vi "I2C Settings from ini.vi"(7 "Section":string, 8 "error in (no error)":errorcluster, 11 "Protocol_Timing In":T1={"SCL Period (Ticks)"=400, "StartDelay(Ticks)"=1200, "StopDelay(Ticks)"=1200, "PostAddressDelay(Ticks)"=1200, "TransmitDelay(Ticks)"=1000}) -> (0 "error out":errorcluster, 3 "Protocol_Timing Out":T1={"SCL Period (Ticks)"=400, "StartDelay(Ticks)"=1200, "StopDelay(Ticks)"=1200, "PostAddressDelay(Ticks)"=1200, "TransmitDelay(Ticks)"=1000}, 5 "All Tags Exists?":bool)   [LabVIEW 2013]
doc: "Loads the I2C Timing protocol parameters from the ini file."
uses:
  Common/File IO/INI/Read write mode.ctl
  I2C Settings Enum Keys.ctl
  I2C/i2c_Protocol_Timing.ctl
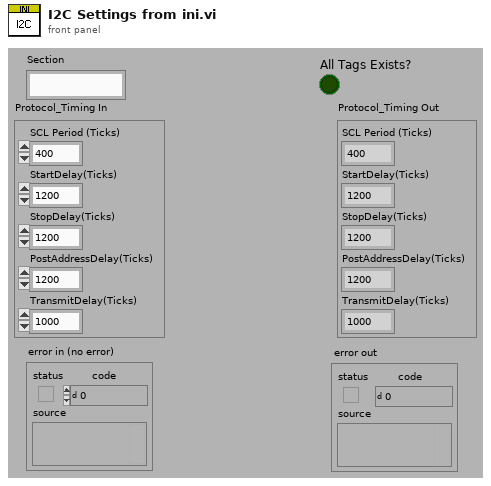
[diagram p1: front panel]
types:
  T1 = typedef "i2c_Protocol_Timing.ctl" = cluster{"SCL Period (Ticks)":u32, "StartDelay(Ticks)":u32, "StopDelay(Ticks)":u32, "PostAddressDelay(Ticks)":u32, "TransmitDelay(Ticks)":u32}
  T2 = typedef "I2C Settings Enum Keys.ctl" = enum16{"SCL Period (Ticks)", "Start Delay (Ticks)", "Stop Delay (Ticks)", "Post Address Delay (Ticks)", "Transmit Delay (Ticks)"}
  T3 = typedef "Read write mode.ctl" = enum16{"Read", "Write"}
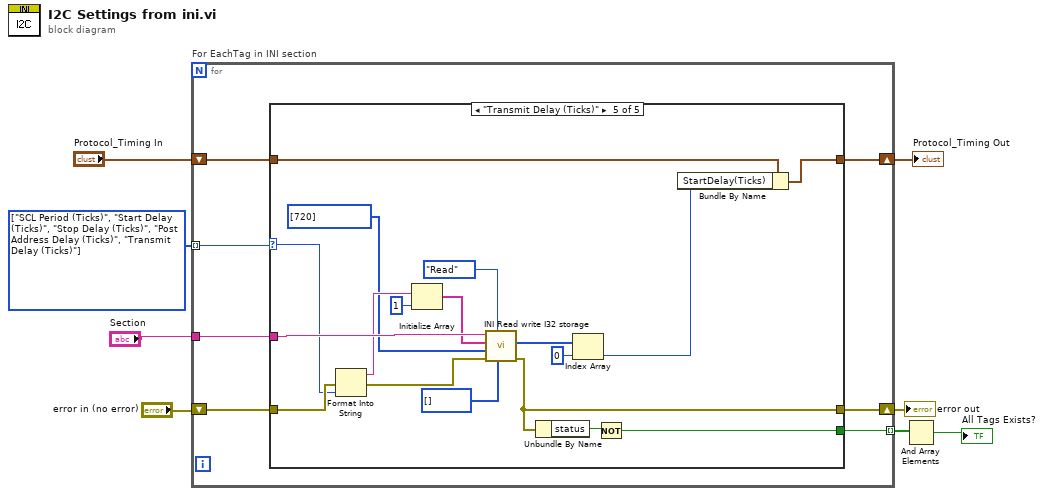
[diagram p0: block diagram]
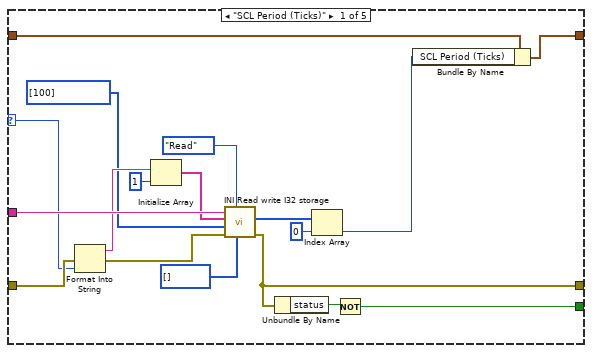
[diagram p2: hidden frame]
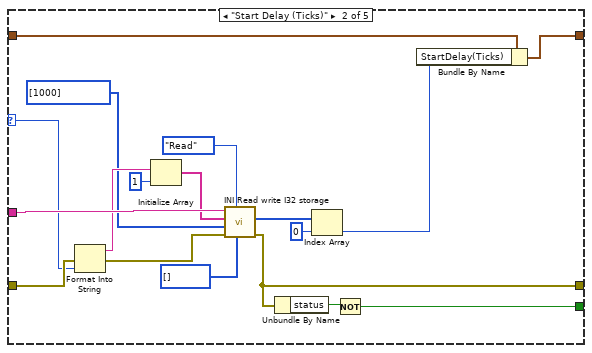
[diagram p3: hidden frame]
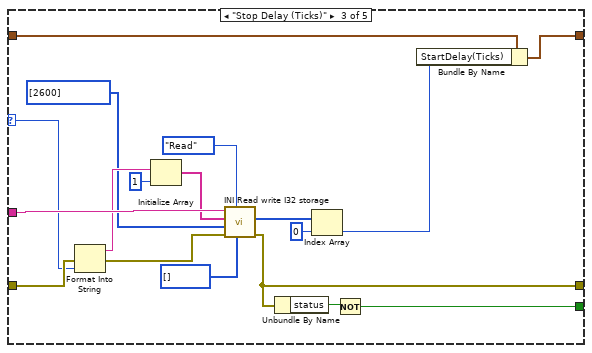
[diagram p4: hidden frame]
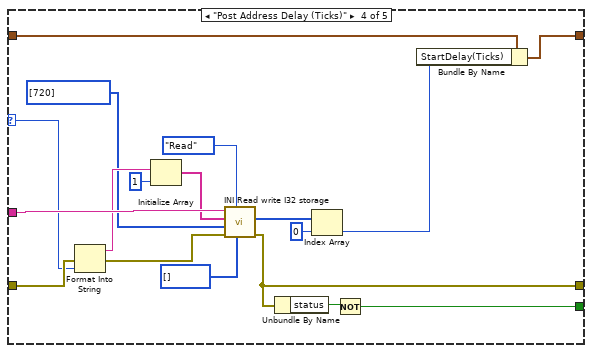
[diagram p5: hidden frame]
diagram:
  w8 = T2[] [enum."SCL Period (Ticks)", enum."Start Delay (Ticks)", enum."Stop Delay (Ticks)", enum."Post Address Delay (Ticks)", enum."Transmit Delay (Ticks)"] items=["SCL Period (Ticks)", "Start Delay (Ticks)", "Stop Delay (Ticks)", "Post Address Delay (Ticks)", "Transmit Delay (Ticks)"]
  n1 = for "For EachTag in INI section" {
    tunnel: "Section" -> [w15]
    tunnel: w8 -> [w14] mode=indexing
    shift-right: [w10] -> w6
    shift-left: "error in (no error)" -> [w12]
    shift-right: [w9] -> w1
    shift-left: "Protocol_Timing In" -> [w13]
    tunnel: [w11] -> w4 mode=indexing
    n2 = case shown="\"Transmit Delay (Ticks)\"" w14 {
      selector: w14 -> [w28 w46 w64 w82 w100]
      tunnel: w15 -> [w32 w50 w68 w86 w104]
      tunnel: w13 -> [w30 w48 w66 w84 w102]
      tunnel: w12 -> [w29 w47 w65 w83 w101]
      tunnel: [w33 w51 w69 w87 w105] -> w10
      tunnel: [w18 w36 w54 w72 w90] -> w11
      tunnel: [w31 w49 w67 w85 w103] -> w9
      frame "SCL Period (Ticks)" {
        n3 = Format Into String(error in=w29, w28) -> (resulting string=w26:string, error out=w19:errorcluster)  [unwired: 2 in]
        n4 = Initialize Array(w26, 1 ("dimension size")) -> (w24:string[])
        n5 = call "INI Read write I32 storage.vi"("Values to write"=i32[] [], "Read/Write mode"=Read_write_mode."Read", "error in"=w19, "Defaults"=i32[] [100], "keys"=w24, "section"=w32) -> ("error out"=w33:errorcluster, "Values"=w23:i32[])  [unwired: 4 in]
        n6 = Unbundle By Name(w33) -> ("status"=w21:bool)
        n7 = Index Array(array=w23, index=0) -> (element=w16:i32)
        n8 = Not(x=w21) -> (.not. x?=w18:bool)
        n9 = Bundle By Name(cluster=w30, "SCL Period (Ticks)"=w16) -> (w31:T1)
      }
      frame "Start Delay (Ticks)" {
        n10 = Format Into String(error in=w47, w46) -> (resulting string=w44:string, error out=w37:errorcluster)  [unwired: 2 in]
        n11 = Initialize Array(w44, 1 ("dimension size")) -> (w42:string[])
        n12 = call "INI Read write I32 storage.vi"("Values to write"=i32[] [], "Read/Write mode"=Read_write_mode."Read", "error in"=w37, "Defaults"=i32[] [1000], "keys"=w42, "section"=w50) -> ("error out"=w51:errorcluster, "Values"=w41:i32[])  [unwired: 4 in]
        n13 = Unbundle By Name(w51) -> ("status"=w39:bool)
        n14 = Index Array(array=w41, index=0) -> (element=w34:i32)
        n15 = Not(x=w39) -> (.not. x?=w36:bool)
        n16 = Bundle By Name(cluster=w48, "StartDelay(Ticks)"=w34) -> (w49:T1)
      }
      frame "Stop Delay (Ticks)" {
        n17 = Format Into String(error in=w65, w64) -> (resulting string=w62:string, error out=w55:errorcluster)  [unwired: 2 in]
        n18 = Initialize Array(w62, 1 ("dimension size")) -> (w60:string[])
        n19 = call "INI Read write I32 storage.vi"("Values to write"=i32[] [], "Read/Write mode"=Read_write_mode."Read", "error in"=w55, "Defaults"=i32[] [2600], "keys"=w60, "section"=w68) -> ("error out"=w69:errorcluster, "Values"=w59:i32[])  [unwired: 4 in]
        n20 = Unbundle By Name(w69) -> ("status"=w57:bool)
        n21 = Index Array(array=w59, index=0) -> (element=w52:i32)
        n22 = Not(x=w57) -> (.not. x?=w54:bool)
        n23 = Bundle By Name(cluster=w66, "StartDelay(Ticks)"=w52) -> (w67:T1)
      }
      frame "Post Address Delay (Ticks)" {
        n24 = Format Into String(error in=w83, w82) -> (resulting string=w80:string, error out=w73:errorcluster)  [unwired: 2 in]
        n25 = Initialize Array(w80, 1 ("dimension size")) -> (w78:string[])
        n26 = call "INI Read write I32 storage.vi"("Values to write"=i32[] [], "Read/Write mode"=Read_write_mode."Read", "error in"=w73, "Defaults"=i32[] [720], "keys"=w78, "section"=w86) -> ("error out"=w87:errorcluster, "Values"=w77:i32[])  [unwired: 4 in]
        n27 = Unbundle By Name(w87) -> ("status"=w75:bool)
        n28 = Index Array(array=w77, index=0) -> (element=w70:i32)
        n29 = Not(x=w75) -> (.not. x?=w72:bool)
        n30 = Bundle By Name(cluster=w84, "StartDelay(Ticks)"=w70) -> (w85:T1)
      }
      frame "Transmit Delay (Ticks)" {
        n31 = Format Into String(error in=w101, w100) -> (resulting string=w98:string, error out=w91:errorcluster)  [unwired: 2 in]
        n32 = Initialize Array(w98, 1 ("dimension size")) -> (w96:string[])
        n33 = call "INI Read write I32 storage.vi"("Values to write"=i32[] [], "Read/Write mode"=Read_write_mode."Read", "error in"=w91, "Defaults"=i32[] [720], "keys"=w96, "section"=w104) -> ("error out"=w105:errorcluster, "Values"=w95:i32[])  [unwired: 4 in]
        n34 = Unbundle By Name(w105) -> ("status"=w93:bool)
        n35 = Index Array(array=w95, index=0) -> (element=w88:i32)
        n36 = Not(x=w93) -> (.not. x?=w90:bool)
        n37 = Bundle By Name(cluster=w102, "StartDelay(Ticks)"=w88) -> (w103:T1)
      }
    }
  }
  "error out" <- w6
  "Protocol_Timing Out" <- w1
  n38 = And Array Elements(Boolean array=w4) -> (logical AND=→"All Tags Exists?":bool)
